vi "Axis String to Enum.vi"(8 "error in (no error)":errorcluster, 10 "Axis String In":string) -> (0 "error out":errorcluster, 2 "Axis Enum Out":T1=enum."A")   [LabVIEW 2017, in "Drivers.lvlib" / "ASI TG-1000.lvlib"]
uses:
  ASI TG-1000.lvlib
  Axis Name.ctl
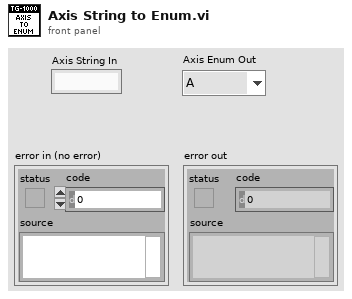
[diagram p1: front panel]
types:
  T1 = typedef "Drivers.lvlib/ASI TG-1000.lvlib/Axis Name.ctl" = enum8{"undefined", "A", "B", "C", "D", "E", "F", "G", "H", "I", "J", "K", "L", "M", "N", "O", "P", "Q", "R", "S", "T", "U", "V", "W", "X", "Y", "Z"}
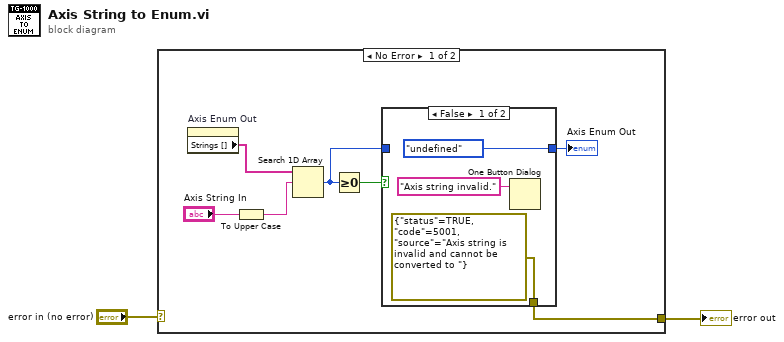
[diagram p0: block diagram]
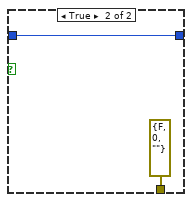
[diagram p2: hidden frame]
diagram:
  n1 = case shown="No Error" "error in (no error)" {
    selector: "error in (no error)" -> [_ w15]
    tunnel: [w3 w15] -> w1
    frame No Error {
      n2 = property on="Axis Enum Out" class="Enum (strict)"() -> ("Strings []"=w8:string[])  [unwired: 2 in, 2 out]
      n3 = To Upper Case(1:"Axis String In") -> (0:w7:string)
      n4 = Search 1D Array(1D array=w8, element=w7) -> (index of element=w5:i32)  [unwired: 1 in]
      n5 = Greater Or Equal To 0?(x=w5) -> (x >= 0?=w6:bool)
      n6 = case shown="False" w6 {
        tunnel: w5 -> [_ w14]
        tunnel: [Axis_Name."undefined" ("Axis Enum Out 2") w14] -> w4
        tunnel: [errorcluster {"status"=TRUE, "code"=5001, "source"="Axis string is invalid and cannot be converted to enum."} ("error constant") errorcluster {"status"=FALSE, "code"=0, "source"=""} ("error constant")] -> w3
        frame False {
          n7 = One Button Dialog(message="Axis string invalid.") -> ()  [unwired: 1 in, 1 out]
        }
        frame True {
        }
      }
      "Axis Enum Out" <- w4
    }
    frame Error {
    }
  }
  "error out" <- w1
